vi "Incoming Events.vi"(11 "ElementEditorPanel in":refnum<class "ElementEditorPanel.lvclass">) -> (2 "Incoming Events":T1, 3 "ElementEditorPanel out":refnum<class "ElementEditorPanel.lvclass">)   [LabVIEW 2020, in "VolatusGUIEditorCore.lvlib" / "ElementEditorPanel.lvclass"]
uses:
  ElementEditorPanel.lvclass
  Incoming Events.ctl
  Update Control Data.ctl
  ElementEditorPanel.lvclass/ElementEditorPanel.ctl
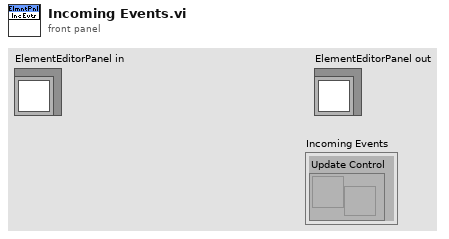
[diagram p1: front panel]
types:
  T1 = typedef "VolatusGUIEditorCore.lvlib/ElementEditorPanel.lvclass/Incoming Events.ctl" = cluster{"Update Control":refnum<user-event>}
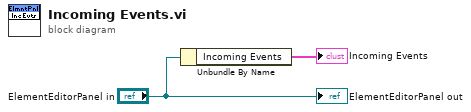
[diagram p0: block diagram]
diagram:
  n1 = Unbundle By Name("ElementEditorPanel in") -> ("Incoming Events"=→"Incoming Events":T1)
  "ElementEditorPanel out" <- "ElementEditorPanel in"
